vi "Initialize MCP.vi"(8 "error in (no error)":errorcluster, 11 "Data Cluster in":T1) -> (0 "error out":errorcluster, 3 "Data Cluster out":T1)   [LabVIEW 2025, in "DQMH MCP Server.lvlib"]
uses:
  DQMH MCP Server.lvlib
  <vilib>/jgoebel/LabVIEW MCP Server SDK/MCP Server.lvlib
  Module Data--cluster.ctl
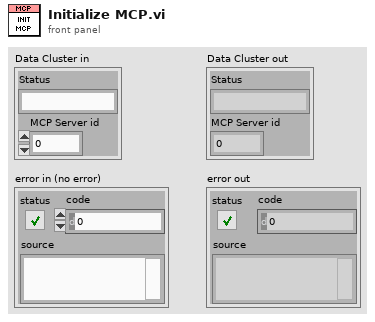
[diagram p1: front panel]
types:
  T1 = typedef "DQMH MCP Server.lvlib/Module Data--cluster.ctl" = cluster{"Status":string, "MCP Server id":i32}
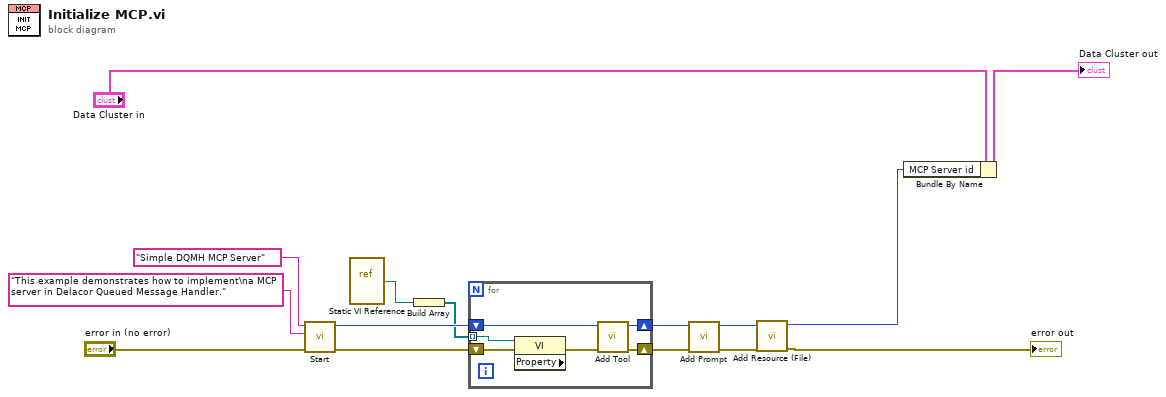
[diagram p0: block diagram]
diagram:
  n1 = call <vilib>:"Start.vi"("error in (no error)"="error in (no error)", "Description"="This example demonstrates how to implement\na MCP server in Delacor Queued Message Handler.", "Name"="Simple DQMH MCP Server") -> ("error out"=w12:errorcluster, "server id out"=w13:i32)  [unwired: 6 in, 1 out]
  n2 = vi-ref "Static VI Reference"() -> ("vi reference"=w2:refnum<vi>)
  n3 = Build Array(w2) -> (w1:refnum<vi>[])
  n4 = for {
    shift-right: [w19] -> w11
    shift-left: w13 -> [w21]
    shift-right: [w18] -> w10
    shift-left: w12 -> [w20]
    tunnel: w1 -> [w16] mode=indexing
    n5 = property class="VI" props=[](reference=w16, error in=w20) -> (error out=w17:errorcluster)  [unwired: 2 out]
    n6 = call <vilib>:"Add Tool.vi"("error in (no error)"=w17, "server id"=w21) -> ("error out"=w18:errorcluster, "server id out"=w19:i32)  [unwired: 8 in]
  }
  n7 = call <vilib>:"Add Prompt.vi"("error in (no error)"=w10, "server id"=w11) -> ("error out"=w8:errorcluster, "server id out"=w9:i32)  [unwired: 8 in]
  n8 = call <vilib>:"Add Resource (File).vi"("error in (no error)"=w8, "server id"=w9) -> ("error out"=→"error out":errorcluster, "server id out"=w3:i32)  [unwired: 8 in]
  n9 = Bundle By Name(cluster="Data Cluster in", "MCP Server id"=w3) -> (→"Data Cluster out":T1)
